vi "iRobot Navigation Target.vi"() -> ()   [LabVIEW 2015]
uses:
  iRobot Sensors.ctl
  iRobot Navigation State Machine.lvsc/StatechartState.ctl
  iRobot Navigation State Machine.lvsc/State.ctl
  iRobot Navigation State Machine.lvsc/Inputs.ctl
  Accelerometer.ctl
  iRobot/Sensor/Sensor Group 6.ctl
  iRobot/Sensor/Bumps + Wheel Drops.ctl
  iRobot/Sensor/Low-Side Driver + Wheel Overcurrent.ctl
  iRobot/Sensor/Buttons.ctl
  iRobot/Sensor/Charging State.ctl
  iRobot/Sensor/Cargo Bay Digital Inputs.ctl
  iRobot/Sensor/Charging Sources Available.ctl
  iRobot/Sensor/OI Mode.ctl
  iRobot Navigation State Machine.lvsc/CompanionDiagram.vi/40/SC Main.vi
  iRobot Navigation State Machine.lvsc/CompanionDiagram.vi/40/Upd State.vi
  iRobot Navigation State Machine.lvsc/CompanionDiagram.vi/40/Trans Graph0.vi
  iRobot Navigation State Machine.lvsc/CompanionDiagram.vi/40/EnterGraphCore.vi
  <vilib>/myRIO/Common/Instrument Driver Framework/myRIO v1.0/UART/vis/myRIO v1.0 Close UART.vi
  iRobot Navigation State Machine.lvsc/CompanionDiagram.vi/40/Trans Graph1.vi
  iRobot Navigation State Machine.lvsc/CompanionDiagram.vi/40/Trans Graph2.vi
  <vilib>/myRIO/Common/Instrument Driver Framework/myRIO v1.0/myRIO v1.1 Open.vi
  iRobot Navigation State Machine.lvsc/CompanionDiagram.vi
  <vilib>/addons/control/pid/pid.llb/PID.vi
  <vilib>/addons/control/pid/pid.llb/PID (DBL).vi
  <vilib>/myRIO/Common/Instrument Driver Framework/Utilities/vis/FPGA Ref Manager.vi
  <vilib>/myRIO/Common/Instrument Driver Framework/myRIO v1.0/myRIO v1.0 Reset FPGA.vi
  <vilib>/myRIO/Common/Instrument Driver Framework/myRIO v1.0/IRQ/vis/myRIO v1.0 IRQ Info FGV.vi
  <vilib>/myRIO/Common/Instrument Driver Framework/myRIO v1.0/IRQ/vis/myRIO v1.0 Timer IRQ Info FGV.vi
  <vilib>/myRIO/Common/Instrument Driver Framework/myRIO v1.0/IRQ/vis/myRIO v1.0 ISR Agent.vi
  iRobot Navigation State Machine.lvsc/Trigger.ctl
  <vilib>/Statechart/Infrastructure/RTStatechart/RunTime SCN.xnode
  iRobot Navigation State Machine.lvsc/Outputs.ctl
  iRobot Navigation State Machine.lvsc
  <vilib>/myRIO/Instrument Drivers/Utilities/Utilities.lvlib
panel:
  in  "Tab Control":T1(tab)
  in  "Kd Constant":dbl
  in  "Ki Constant":dbl=30.0
  in  "Kp Constant":dbl=350.0
  out "Right wheel":i16
  out "Left wheel":i16
  out "PID output":dbl
  out "iRobot Sensors (graphical)":T2 {"Right Wheel (mm/s)" scale=-500.0..500.0; "Left Wheel (mm/s)" scale=-500.0..500.0}
  out "Active States":T4
  out "error out":errorcluster
  in  "Wheel Speed (mm/s)":i16(slide)=100 scale=0.0..500.0
  in  "accel smoothing (0-1)":dbl=0.1
  in  "stop":bool
  out "Target Running":bool
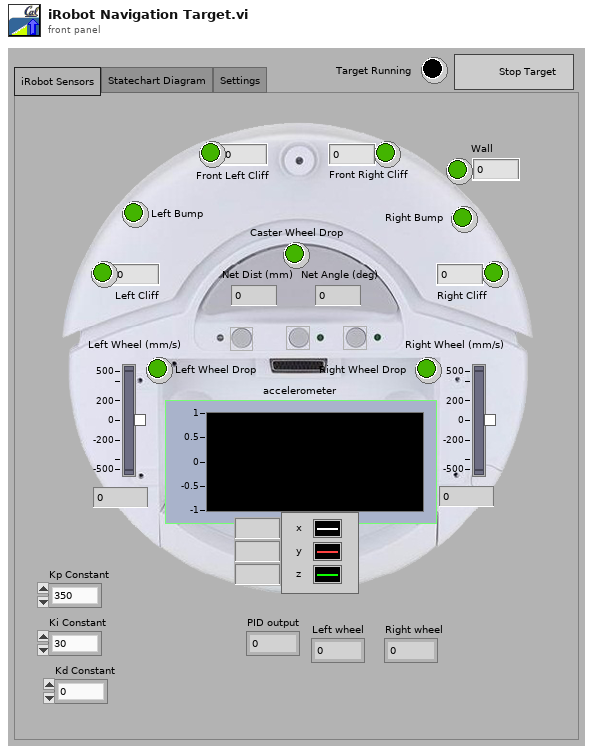
[diagram p1: front panel]
types:
  T1 = enum32{"iRobot Sensors", "Statechart Diagram", "Settings"}
  T2 = typedef "iRobot Sensors.ctl" = cluster{"Caster Wheel Drop":bool, "Left Wheel Drop":bool, "Right Wheel Drop":bool, "Left Bump":bool, "Right Bump":bool, "Left Cliff":bool, "Front Left Cliff":bool, "Front Right Cliff":bool, "Right Cliff":bool, "Wall":bool, "Net Dist (mm)":i32, "Net Angle (deg)":i32, "Wall":u16, "Left Cliff":u16, "Front Left Cliff":u16, "Front Right Cliff":u16, "Right Cliff":u16, "Left Wheel (mm/s)":i16, "Right Wheel (mm/s)":i16, "accelerometer":T3}
  T3 = typedef "Accelerometer.ctl" = cluster{"x axis (g)":dbl, "y axis (g)":dbl, "z axis (g)":dbl}
  T4 = typedef "iRobot Navigation State Machine.lvsc/StatechartState.ctl" = T5[]
  T5 = typedef "iRobot Navigation State Machine.lvsc/State.ctl" = enum16{"NI.SC.Initial", "NI.SC.History", "NI.SC.ShallowHistory", "NI.SC.Terminal", "Pause", "Run", "Pause\\Detect Play Button\\Pause;\nWait for\nbutton\nrelease", "Pause\\Detect Play Button\\Unpause;\nwait for\nbutton release", "Pause\\Detect Play Button\\Unpause;\nwait for\nbutton press", "Run\\Detect Obstacles\\Right Bumper", "Run\\Detect Obstacles\\Left Bumper", "Run\\Detect Obstacles\\Turn Right", "Run\\Detect Obstacles\\Turn Left", "Run\\Detect Obstacles\\Drive"}
  T6 = typedef "iRobot UART Port Type.ctl" = refnum<visa-resource-name>
  T7 = typedef "iRobot Navigation State Machine.lvsc/Inputs.ctl" = cluster{"net distance (mm)":i32, "net angle (deg)":i32, "Max Wheel Speed (mm/s)":i16, "accelerometer":T3, "iRobot Sensors":T8, "Is Simulator?":bool, "Kp Constant":dbl, "Ki Constant":dbl, "Kd Constant":dbl}
  T8 = typedef "Sensor Group 6.ctl" = cluster{"Bumps + Wheel Drops":T9, "Wall":bool, "Cliff Left":bool, "Cliff Front Left":bool, "Cliff Front Right":bool, "Cliff Right":bool, "Virtual Wall":bool, "Low-Side Driver + Wheel Overcurrent":T10, "Infrared":u8, "Buttons":T11, "Distance (mm)":i32, "Angle (deg)":i32, "Charging State":T12, "Voltage (mV)":u16, "Current (mA)":i16, "Battery Temperature (deg C)":i8, "Battery Charge (mAh)":u16, "Battery Capacity (mAh)":u16, "Wall Signal (0-4095)":u16, "Cliff Left Signal (0-4095)":u16, "Cliff Front Left Signal (0-4095)":u16, "Cliff Front Right Signal (0-4095)":u16, "Cliff Right Signal (0-4095)":u16, "Cargo Bay Digital Inputs":T13, "Cargo Bay Analog Signal (0-1023)":u16, "Charging Sources Available":T14, "OI Mode":T15, "Song Number":u8, "Song Playing":bool, "Number of Stream Packets":u8, "Requested Velocity (mm/s)":i16, "Requested Radius (mm)":i16, "Requested Right Wheel Velocity (mm/s)":i16, "Requested Left Wheel Velocity (mm/s)":i16}
  T9 = typedef "Bumps + Wheel Drops.ctl" = cluster{"Wheeldrop Caster":bool, "Wheeldrop Left":bool, "Wheeldrop Right":bool, "Bump Left":bool, "Bump Right":bool}
  T10 = typedef "Low-Side Driver + Wheel Overcurrent.ctl" = cluster{"Low-Side Driver 0":bool, "Low-Side Driver 1":bool, "Low-Side Driver 2":bool, "Left Wheel":bool, "Right Wheel":bool}
  T11 = typedef "Buttons.ctl" = cluster{"Advance":bool, "Play":bool}
  T12 = typedef "Charging State.ctl" = enum16{"Not Charging", "Reconditioning Charging", "Full Charging", "Trickle Charging", "Waiting", "Charging Fault Condition"}
  T13 = typedef "Cargo Bay Digital Inputs.ctl" = cluster{"Digital Input 0":bool, "Digital Input 1":bool, "Digital Input 2":bool, "Digital Input 3":bool, "Device Detect":bool}
  T14 = typedef "Charging Sources Available.ctl" = cluster{"Internal Charger":bool, "Home Base":bool}
  T15 = typedef "OI Mode.ctl" = enum16{"Off", "Passive", "Safe", "Full"}
  T16 = typedef "iRobot Navigation State Machine.lvsc/Outputs.ctl" = cluster{"Left Wheel Speed (mm/s)":i16, "Right Wheel Speed (mm/s)":i16, "PID output":dbl, "Left Wheel":i16, "Right Wheel":i16}
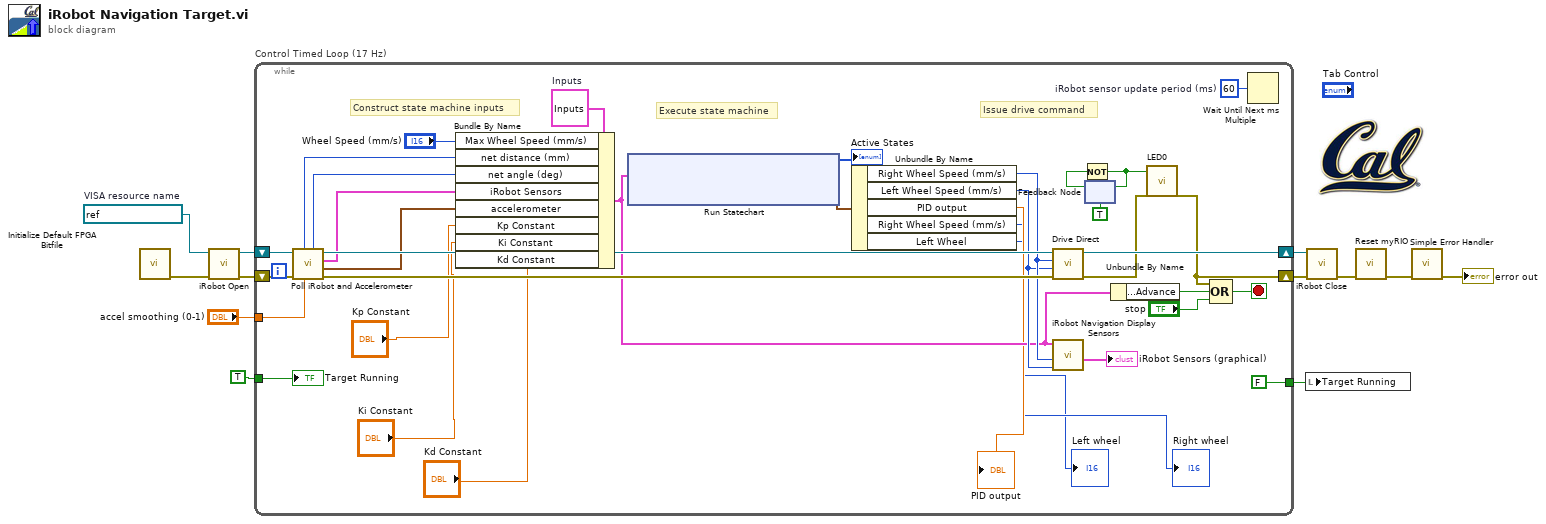
[diagram p0: block diagram]
diagram:
  w6 = refnum<visa-resource-name> "ASRL1::INSTR"  # VISA resource name
  n1 = call <vilib>:"Initialize Default FPGA Bitfile.vi"() -> ("error out"=w4:errorcluster)  [unwired: 11 in]
  n2 = call "iRobot Open.vi"("error in (no error)"=w4, "UART port in"=w6) -> ("error out"=w11:errorcluster, "UART port out"=w10:T6)  [unwired: 8 in]
  n3 = while "Control Timed Loop (17 Hz)" {
    shift-right: [w47] -> w12
    shift-left: w10 -> [w42]
    shift-right: [w29] -> w7
    shift-left: w11 -> [w41]
    tunnel: TRUE ("stop") -> [w35]
    tunnel: [FALSE ("stop")] -> w8
    tunnel: "accel smoothing (0-1)" -> [w21]
    stop <- w46 stop-if-true
    w19 = u32 60  # iRobot sensor update period (ms)
    w44 = T7 {"net distance (mm)"=0, "net angle (deg)"=0, "Max Wheel Speed (mm/s)"=0, "accelerometer"={"x axis (g)"=0.0, "y axis (g)"=0.0, "z axis (g)"=0.0}, "iRobot Sensors"={"Bumps + Wheel Drops"={"Wheeldrop Caster"=FALSE, "Wheeldrop Left"=FALSE, "Wheeldrop Right"=FALSE, "Bump Left"=FALSE, "Bump Right"=FALSE}, "Wall"=FALSE, "Cliff Left"=FALSE, "Cliff Front Left"=FALSE, "Cliff Front Right"=FALSE, "Cliff Right"=FALSE, "Virtual Wall"=FALSE, "Low-Side Driver + Wheel Overcurrent"={"Low-Side Driver 0"=FALSE, "Low-Side Driver 1"=FALSE, "Low-Side Driver 2"=FALSE, "Left Wheel"=FALSE, "Right Wheel"=FALSE}, "Infrared"=255, "Buttons"={"Advance"=FALSE, "Play"=FALSE}, "Distance (mm)"=0, "Angle (deg)"=0, "Charging State"=enum."Not Charging", "Voltage (mV)"=0, "Current (mA)"=0, "Battery Temperature (deg C)"=0, "Battery Charge (mAh)"=0, "Battery Capacity (mAh)"=0, "Wall Signal (0-4095)"=0, "Cliff Left Signal (0-4095)"=0, "Cliff Front Left Signal (0-4095)"=0, "Cliff Front Right Signal (0-4095)"=0, "Cliff Right Signal (0-4095)"=0, "Cargo Bay Digital Inputs"={"Digital Input 0"=FALSE, "Digital Input 1"=FALSE, "Digital Input 2"=FALSE, "Digital Input 3"=FALSE, "Device Detect"=FALSE}, "Cargo Bay Analog Signal (0-1023)"=0, "Charging Sources Available"={"Internal Charger"=FALSE, "Home Base"=FALSE}, "OI Mode"=enum."Off", "Song Number"=0, "Song Playing"=FALSE, "Number of Stream Packets"=0, "Requested Velocity (mm/s)"=0, "Requested Radius (mm)"=0, "Requested Right Wheel Velocity (mm/s)"=0, "Requested Left Wheel Velocity (mm/s)"=0}, "Is Simulator?"=FALSE, "Kp Constant"=0.0, "Ki Constant"=0.0, "Kd Constant"=0.0}  # Inputs
    # "Issue drive command"
    # "Execute state machine"
    # "Construct state machine inputs"
    n4 = call "Poll iRobot and Accelerometer.vi"("accel smoothing (0-1)"=w21, "error in"=w41, "UART port in"=w42) -> ("error out"=w40:errorcluster, "Acceleration (g)"=w20:T3, "iRobot SensorGroup6"=w28:T8, "UART port out"=w39:T6, "net angle (deg)"=w37:i32, "net distance (mm)"=w38:i32)  [unwired: 3 in]
    n5 = Bundle By Name(cluster=w44, "Max Wheel Speed (mm/s)"="Wheel Speed (mm/s)", "net distance (mm)"=w38, "net angle (deg)"=w37, "iRobot Sensors"=w28, "accelerometer"=w20, "Kp Constant"="Kp Constant", "Ki Constant"="Ki Constant", "Kd Constant"="Kd Constant") -> (w23:T7)
    n6 = xnode "Run Statechart"("Inputs"=w23) -> ("Outputs"=w45:T16, "Active States"=→"Active States":T4)  [unwired: 2 in, 1 out]
    n7 = Unbundle By Name(w45) -> ("Right Wheel Speed (mm/s)"=w26:i16, "Left Wheel Speed (mm/s)"=w25:i16, "PID output"=→"PID output":dbl, "Right Wheel Speed (mm/s)"=→"Right wheel":i16, "Left Wheel"=→"Left wheel":i16)
    n8 = call "Drive Direct.vi"("error in"=w40, "Left Wheel Velocity (mm/s)"=w25, "Right Wheel Velocity (mm/s)"=w26, "UART port in"=w39) -> ("error out"=w30:errorcluster, "UART port out"=w47:T6)  [unwired: 6 in]
    n9 = call "iRobot Navigation Display Sensors.vi"("Left Wheel (mm/s)"=w25, "Right Wheel (mm/s)"=w26, "Statechart Inputs"=w23) -> ("iRobot Sensors (graphical)"=→"iRobot Sensors (graphical)":T2)  [unwired: 6 in]
    n10 = feedback #1(TRUE) -> (w31:bool)
    n11 = Not(x=w31) -> (.not. x?=w32:bool)
    n12 = feedback-in #1(w32) -> ()
    n13 = Unbundle By Name(w23) -> ("iRobot Sensors.Buttons.Advance"=w22:bool)
    n14 = call "LED0"("LED0"=w32, "error in (no error)"=w30) -> ("error out"=w29:errorcluster)  [unwired: 25 in]
    n15 = Compound Arithmetic op=OR(w29, w22, "stop") -> (w46:bool)
    n16 = Wait Until Next ms Multiple(millisecond multiple=w19) -> ()  [unwired: 1 out]
    "Target Running" <- w35
  }
  n17 = local write "Target Running"(w8) -> ()
  n18 = call "iRobot Close.vi"("error in"=w7, "UART port in"=w12) -> ("error out"=w1:errorcluster)  [unwired: 9 in]
  n19 = call <vilib>:"Reset myRIO.vi"("error in (no error)"=w1) -> ("error out"=w5:errorcluster)  [unwired: 10 in]
  n20 = call <vilib>:"Simple Error Handler.vi"("error in (no error)"=w5) -> ("error out"=→"error out":errorcluster)  [unwired: 4 in, 4 out]
